vi "AI StartStop.vi"(11 "acquire":bool) -> ()   [LabVIEW 2019]
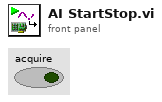
[diagram p1: front panel]
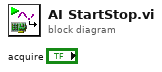
[diagram p0: block diagram]
diagram:
